vi "Imports.vi"(6 "error in":errorcluster, 9 "PythonConverter_BD in":refnum<class "PyConvBD.lvclass">) -> (0 "error out":errorcluster, 3 "PythonConverter_BD out":refnum<class "PyConvBD.lvclass">, 4 "imports":string)   [LabVIEW 2014, in "Raspberry Pi Compatible Compiler for LabVIEW.lvlib" / "PyConvBD.lvclass"]
uses:
  PyConvBD.lvclass
  PyConvBD.lvclass/PyConvBD.ctl
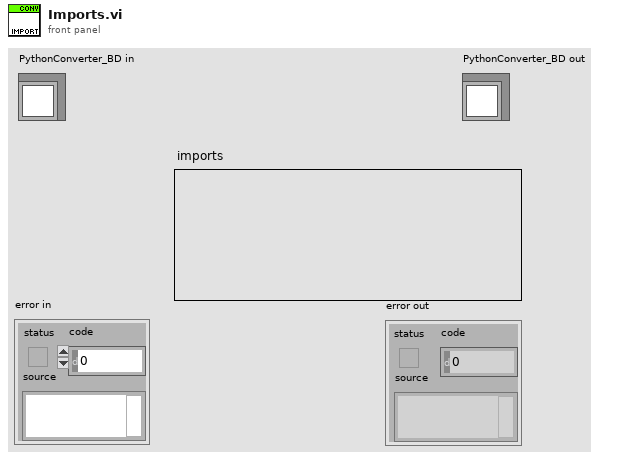
[diagram p1: front panel]
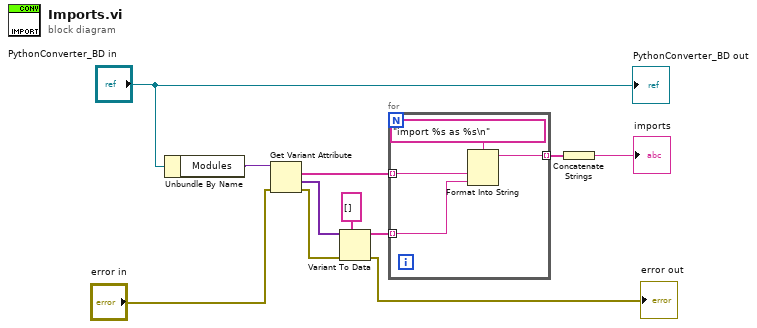
[diagram p0: block diagram]
diagram:
  n1 = Unbundle By Name("PythonConverter_BD in") -> ("Modules"=w4:variant)
  n2 = Get Variant Attribute(Variant=w4, error in="error in") -> (names=w8:string[], values=w5:variant[], error out=w10:errorcluster)  [unwired: 2 in, 1 out]
  n3 = Variant To Data(error in=w10, type=string[] [], Variant=w5) -> (data=w7:string[], error out=→"error out":errorcluster)
  n4 = for {
    tunnel: w7 -> [w14] mode=indexing
    tunnel: w8 -> [w15] mode=indexing
    tunnel: [w12] -> w9 mode=indexing
    n5 = Format Into String(format string="import %s as %s\n", w15, w14) -> (resulting string=w12:string)  [unwired: 2 in, 1 out]
  }
  n6 = Concatenate Strings(w9) -> (→"imports":string)
  "PythonConverter_BD out" <- "PythonConverter_BD in"
